vi "Sm To Dkm.vi"(8 "error in (no error)":errorcluster, 10 "error":i32, 11 "sMetres":string) -> (0 "error out":i32, 1 "error out 2":errorcluster, 2 "dkm":dbl, 3 "sMetres out":string)   [LabVIEW 2023, in "POSCONV.lvlib"]
doc: "Converts string metres to double kilometres (1km = 1000m)...\n\n\ndouble SmToDkm(char *sMetres, int *error);"
uses:
  POSCONV.lvlib
  C:/Users/J Gordon/Documents/Rail Tech/TV-HR/02 - Code/Modules/POSCONV/POSCONV.dll
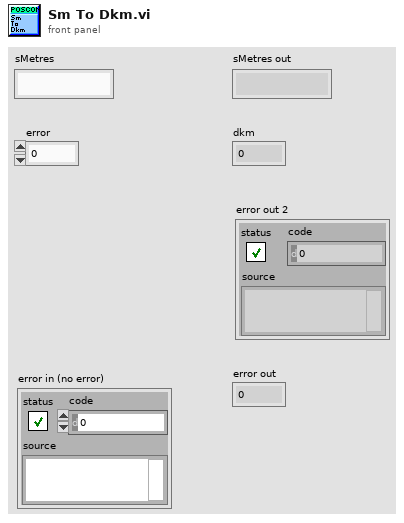
[diagram p1: front panel]
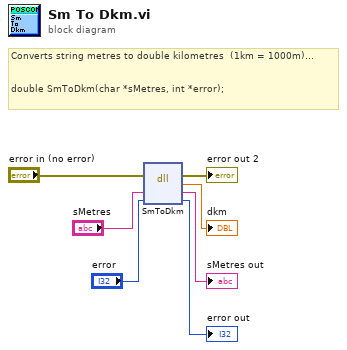
[diagram p0: block diagram]
diagram:
  # "Converts string metres to double kilometres  (1km = 1000m)...\n\n\ndouble SmToDkm(char *sMetres, int *error);"
  n1 = dll-call lib="C:/Users/J Gordon/Documents/Rail Tech/TV-HR/02 - Code/Modules/POSCONV/POSCONV.*" fn="SmToDkm"(error in="error in (no error)", "sMetres"="sMetres", "error"="error") -> (error out=→"error out 2":errorcluster, →"dkm":dbl, "sMetres"=→"sMetres out":string, "error"=→"error out":i32)  [unwired: 2 in, 1 out]
